vi "remove_waveforms.vi"(8 "error in (no error)":errorcluster, 11 "HSDIO in":refnum<class "HSDIO.lvclass">) -> (0 "error out":errorcluster, 3 "HSDIO out":refnum<class "HSDIO.lvclass">)   [LabVIEW 2013, in "HSDIO.lvclass"]
uses:
  HSDIO.lvclass
  HSDIO.lvclass/HSDIO.ctl
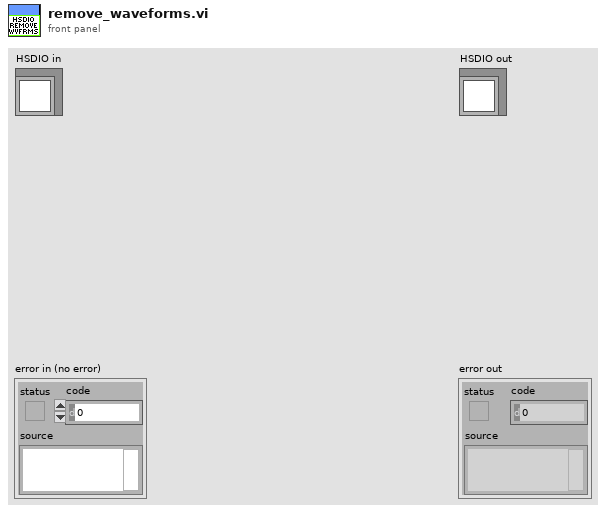
[diagram p1: front panel]
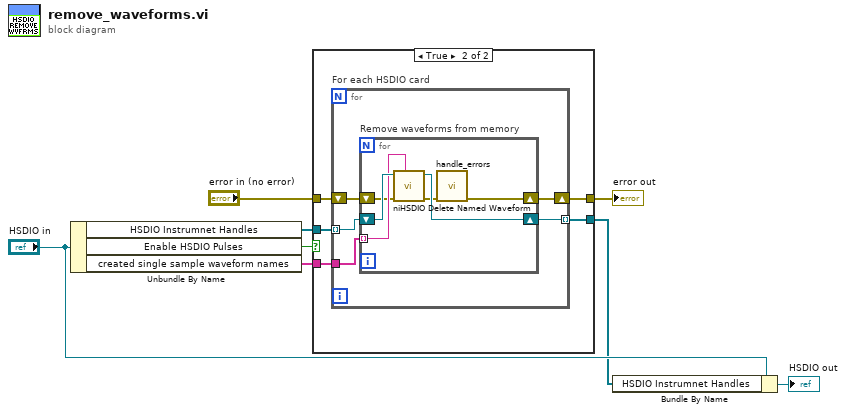
[diagram p0: block diagram]
diagram:
  n1 = Unbundle By Name("HSDIO in") -> ("HSDIO Instrumnet Handles"=w4:refnum<k15>[], "Enable HSDIO Pulses"=w2:bool, "created single sample waveform names"=w1:string[])
  n2 = case shown="True" w2 {
    tunnel: w4 -> [w9 w15]
    tunnel: [w9 w14] -> w3
    tunnel: w1 -> [_ w13]
    tunnel: "error in (no error)" -> [w10 w12]
    tunnel: [w10 w11] -> w7
    frame False {
    }
    frame True {
      n3 = for "For each HSDIO card" {
        tunnel: w15 -> [w20] mode=indexing
        tunnel: [w19] -> w14 mode=indexing
        tunnel: w13 -> [w18]
        shift-right: [w16] -> w11
        shift-left: w12 -> [w17]
        n4 = for "Remove waveforms from memory" {
          shift-right: [w21] -> w16
          shift-left: w17 -> [w23]
          shift-right: [w25] -> w19
          shift-left: w20 -> [w26]
          tunnel: w18 -> [w24] mode=indexing
          n5 = call <instrlib>:"niHSDIO Delete Named Waveform.vi"("waveform name (default:\"\")"=w24, "error in (no error)"=w23, "instrument handle"=w26) -> ("error out"=w22:errorcluster, "instrument handle out"=w25:refnum<k15>)  [unwired: 7 in]
          n6 = call "handle_errors.vi"("error in (no error)"=w22) -> ("error out"=w21:errorcluster)  [unwired: 14 in]
        }
      }
    }
  }
  "error out" <- w7
  n7 = Bundle By Name(cluster="HSDIO in", "HSDIO Instrumnet Handles"=w3) -> (→"HSDIO out":refnum<class "HSDIO.lvclass">)
